vi "File.Get Folder Contents Info.vi"(8 "error in (no error)":errorcluster, 11 "Folder":path) -> (0 "error out":errorcluster, 1 "RelPaths":string[](array[string]), 3 "File Info":T1[](array[typedef]))   [LabVIEW 2024, in "KATE_Lib.lvlib" / "File Utils.lvlib"]
uses:
  File Utils.lvlib
  File.File Compare Info.ctl
  Status/Status Utils.lvlib
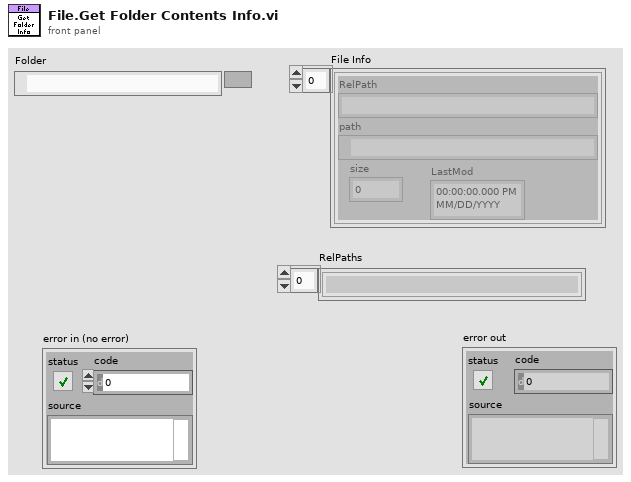
[diagram p1: front panel]
types:
  T1 = typedef "KATE_Lib.lvlib/File Utils.lvlib/File.File Compare Info.ctl" = cluster{"RelPath":string, "path":path, "size":i64, "LastMod":timestamp}
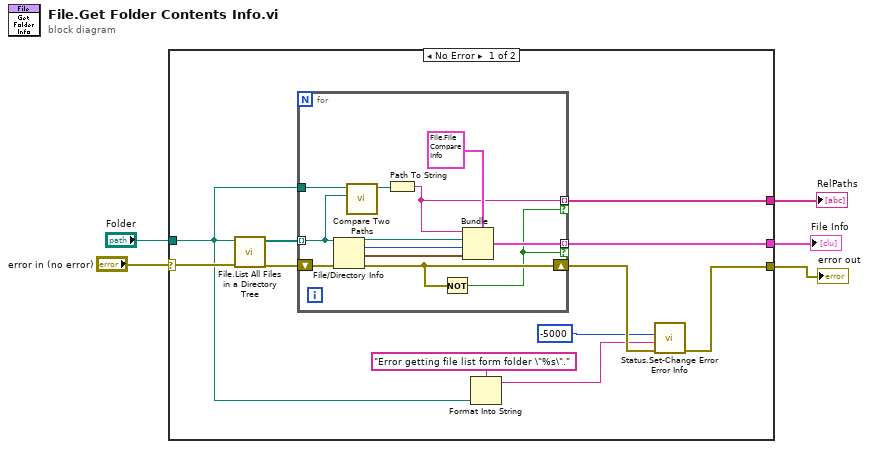
[diagram p0: block diagram]
diagram:
  n1 = case shown="No Error" "error in (no error)" {
    selector: "error in (no error)" -> [w12 w29]
    tunnel: "Folder" -> [w7 _]
    tunnel: [w15 _] -> w4
    tunnel: [w14 _] -> w3
    tunnel: [w10 w29] -> w1
    frame No Error {
      n2 = call "File.List All Files in a Directory Tree.vi"("error in (no error)"=w12, "Folder"=w7) -> ("error out"=w13:errorcluster, "Files"=w16:path[])  [unwired: 8 in]
      n3 = for {
        tunnel: w16 -> [w23] mode=indexing
        tunnel: [w25] -> w15 mode=indexing if=w17
        tunnel: w7 -> [w24]
        tunnel: [w20] -> w14 mode=indexing if=w17
        shift-right: [w18] -> w11
        shift-left: w13 -> [w19]
        n4 = File/Directory Info(path=w23, error in=w19) -> (path out=w28:path, size=w27:i64, last mod=w26:timestamp, error out=w18:errorcluster)  [unwired: 3 out]
        n5 = call <vilib>:"Compare Two Paths.vi"("Path 2"=w23, "Path 1"=w24) -> ("Relative Path from 1 to 2"=w21:path)  [unwired: 6 in, 3 out]
        n6 = Path To String(path=w21) -> (string=w20:string)
        n7 = Not(x=w18) -> (.not. x?=w17:bool)
        n8 = Bundle(cluster=T1 {"RelPath"="", "path"=path "", "size"=0, "LastMod"=timestamp(0 s since 1904-01-01)}, "RelPath"=w20, "path"=w28, "size"=w27, "LastMod"=w26) -> (w25:T1)
      }
      n9 = Format Into String(format string="Error getting file list form folder \"%s\".", w7) -> (resulting string=w6:string)  [unwired: 2 in, 1 out]
      n10 = call "Status.Set-Change Error Error Info.vi"("Error In"=w11, "NewDesc"=w6, "NewCode"=-5000) -> ("Error Out"=w10:errorcluster)  [unwired: 8 in]
    }
    frame Error {
    }
  }
  "File Info" <- w4
  "RelPaths" <- w3
  "error out" <- w1
